vi "一维数组重复数目_字符串.vi"(1 "元素":string, 2 "数组":string[](array[string])) -> (0 "个数":i32)   [LabVIEW 2014]
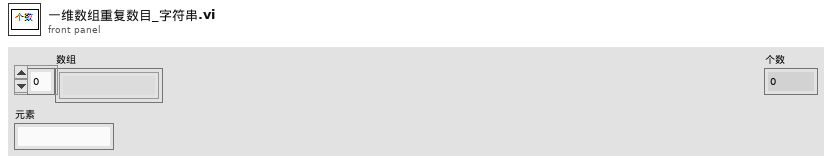
[diagram p1: front panel]
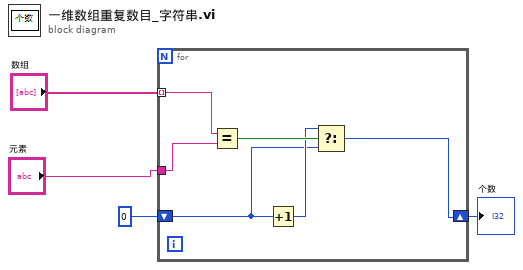
[diagram p0: block diagram]
diagram:
  n1 = for {
    tunnel: "数组" -> [w10] mode=indexing
    tunnel: "元素" -> [w9]
    shift-right: [w5] -> w1
    shift-left: 0 -> [w6]
    n2 = Equal?(x=w10, y=w9) -> (x = y?=w8:bool)
    n3 = Increment(x=w6) -> (x+1=w7:i32)
    n4 = Select(t=w7, s=w8, f=w6) -> (s? t:f=w5:i32)
  }
  "个数" <- w1
